vi "solar_gbl Launch Targets.vi"(7 "Splash VI Refnum":refnum<vi>, 8 "error in (no error)":errorcluster, 10 "Default Targets (name,vi)":string[][](array[string]), 11 "SOLAR in":T1) -> (0 "error out":errorcluster, 2 "TargetVIs":refnum<vi>[](array[refnum]), 3 "SOLAR out":T1)   [LabVIEW 2018]
doc: "This launches the targets specified in the solar.ini configuration file. The target VI must wire the 'Target' string control to the upper left connector pane terminal of the 4-2-2-4 layout. The targets are separated on each line of the 'Targets' configuration key formatted as:\nTargets = 'TARGET,VI\nTARGET,VI\""
uses:
  solar_ctl SOLAR Global.ctl
  solar_ctl Target Global.ctl
  voyager/solar_voy_ctl Voyager Refnum.ctl
  qtimer/solar_qtimer_ctl Refnum.ctl
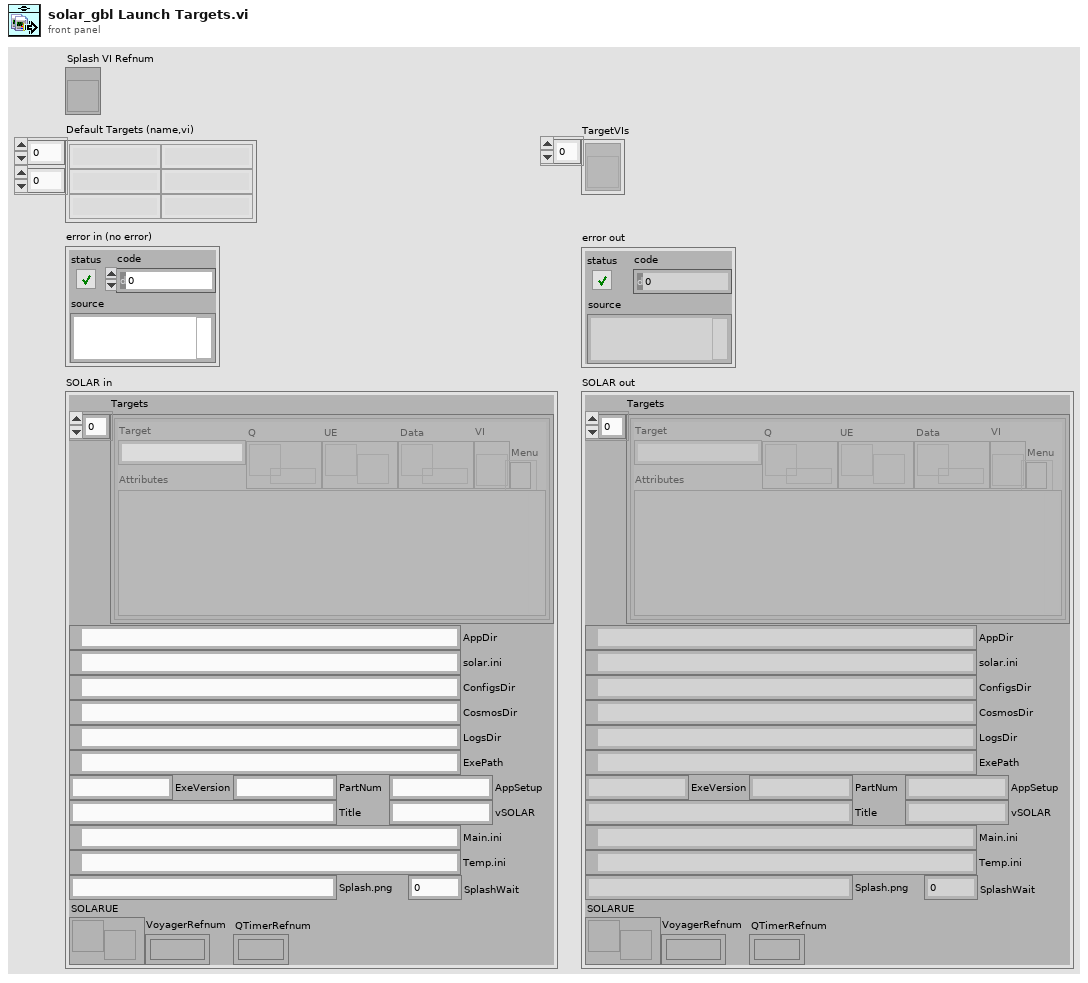
[diagram p1: front panel]
types:
  T1 = typedef "solar_ctl SOLAR Global.ctl" = cluster{"Targets":T2[], "AppDir":path, "solar.ini":path, "ConfigsDir":path, "CosmosDir":path, "LogsDir":path, "ExePath":path, "ExeVersion":string, "PartNum":string, "AppSetup":string, "Title":string, "Main.ini":path, "Temp.ini":path, "vSOLAR":string, "Splash.png":string, "SplashWait":i32, "SOLARUE":refnum<user-event>, "VoyagerRefnum":T3, "QTimerRefnum":T4}
  T2 = typedef "solar_ctl Target Global.ctl" = cluster{"Target":string, "Q":refnum<queue>, "UE":refnum<user-event>, "VI":refnum<vi>, "Menu":refnum<k9>, "Data":refnum<data-value>, "Attributes":variant}
  T3 = typedef "solar_voy_ctl Voyager Refnum.ctl" = refnum<k1>
  T4 = typedef "solar_qtimer_ctl Refnum.ctl" = refnum<k1>
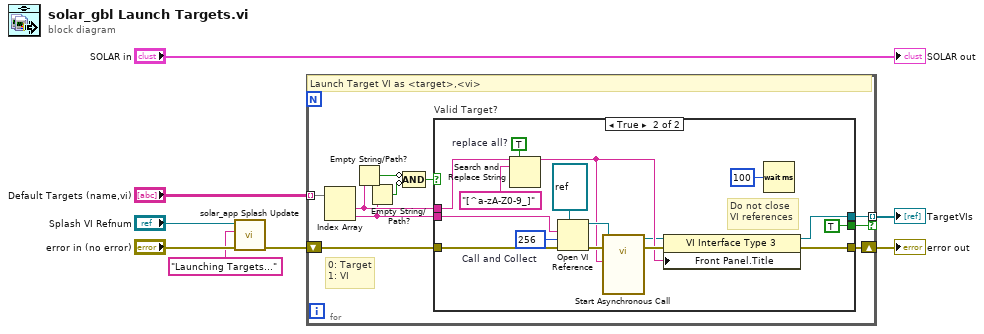
[diagram p0: block diagram]
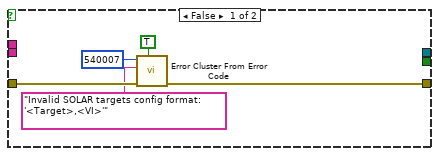
[diagram p2: hidden frame]
diagram:
  n1 = call "solar_app Splash Update.vi"("error in (no error)"="error in (no error)", "Info"="Launching Targets...", "Splash VI Refnum in"="Splash VI Refnum") -> ("error out"=w4:errorcluster)  [unwired: 7 in, 1 out]
  n2 = for {
    shift-right: [w13] -> w7
    shift-left: w4 -> [w14]
    tunnel: "Default Targets (name,vi)" -> [w18] mode=indexing
    tunnel: [w10] -> w1 mode=indexing if=w9
    # "0: Target\n1: VI"
    # "Launch Target VI as <target>,<vi>"
    n3 = Index Array(array=w18) -> (element #1=w12:string, element #2=w11:string)  [unwired: 2 in]
    n4 = Empty String/Path?(string/path=w12) -> (empty?=w15:bool)
    n5 = Empty String/Path?(string/path=w11) -> (empty?=w16:bool)
    n6 = Compound Arithmetic op=AND(invert w15, invert w16) -> (w17:bool)
    n7 = case "Valid Target?" shown="True" w17 {
      tunnel: w14 -> [w23 w34]
      tunnel: [w20 w36] -> w13
      tunnel: w12 -> [_ w37]
      tunnel: w11 -> [_ w32]
      tunnel: [_ w25] -> w10
      tunnel: [_ TRUE] -> w9
      frame False {
        n8 = call <vilib>:"Error Cluster From Error Code.vi"("show call chain? (False)"=TRUE, "error in (no error)"=w23, "error message (\"\")"="Invalid SOLAR targets config format: '<Target>,<VI>'" ("source"), "error code (0)"=540007 ("code")) -> ("error out"=w20:errorcluster)  [unwired: 5 in]
      }
      frame True {
        w31 = 256  # Call and Collect
        w39 = TRUE  # replace all?
        # "Do not close\nVI references"
        n9 = Search and Replace String(replace all?=w39, input string=w37, search string="[^a-zA-Z0-9_]") -> (result string=w27:string)  [unwired: 5 in, 3 out]
        n10 = Open VI Reference(type specifier VI Refnum (for type only)=refnum<vi> refnum, vi path=w32, options=w31, error in (no error)=w34) -> (vi reference=w28:refnum<vi>, error out=w30:errorcluster)  [unwired: 2 in]
        n11 = call-by-ref "Start Asynchronous Call"(reference=w28, error in=w30, "Target"=w27) -> (reference out=w26:refnum<vi>, error out=w29:errorcluster)  [unwired: 11 in]
        n12 = property class="VI Interface Type 3"(reference=w26, error in=w29, "Front Panel.Title"=w27) -> (reference out=w25:refnum<vi>, error out=w36:errorcluster)
        n13 = Wait (ms)(milliseconds to wait=u32 100) -> ()  [unwired: 1 out]
      }
    }
  }
  "error out" <- w7
  "TargetVIs" <- w1
  "SOLAR out" <- "SOLAR in"
